vi "GetBestGuess2.vi"(9 "threshold":dbl=0.6, 10 "APIKey":string, 11 "Image":path=path "/Users/crogers/Desktop/AllThingsLEGO/AI/Ziyi/imageTest") -> (1 "score":dbl, 2 "class":string, 3 "All Data":T1)   [LabVIEW 2019]
uses:
  <vilib>/httpClient/MultipartData.ctl
  <vilib>/httpClient/LabVIEWHTTPClient.lvlib
panel:
  out "Body":string
  out "Headers":string="\r\n\r\n"
  out "error out":errorcluster
  out "Most likely":cluster{"score":dbl, "class":string}[](array[cluster])
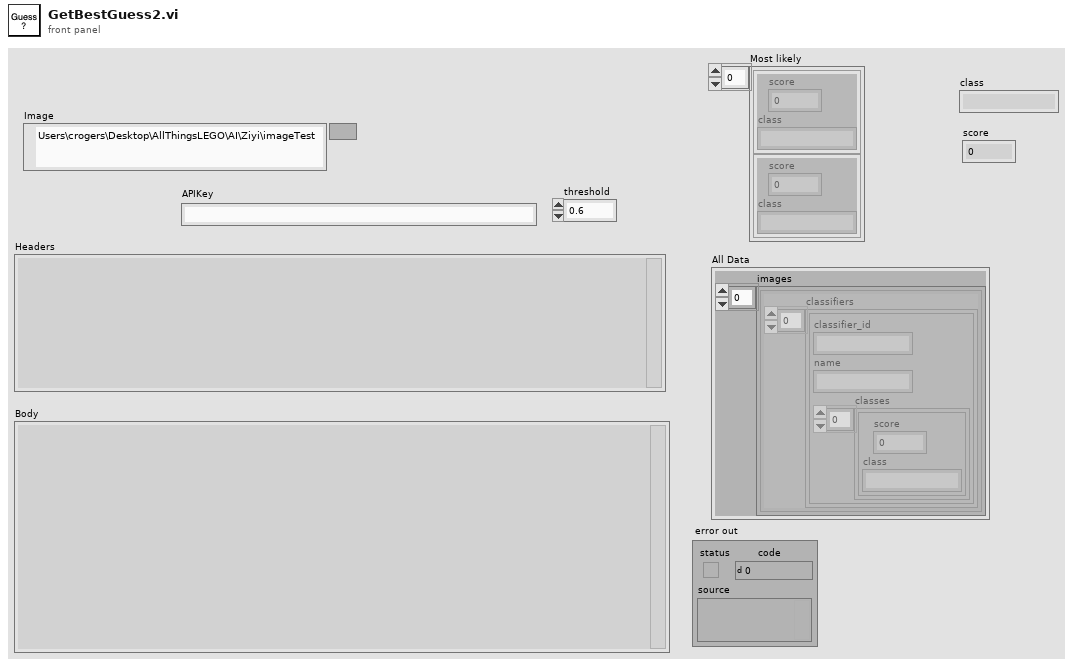
[diagram p1: front panel]
types:
  T1 = cluster{"images":cluster{"classifiers":cluster{"classifier_id":string, "name":string, "classes":cluster{"score":dbl, "class":string}[]}[]}[]}
  T2 = typedef "LabVIEWHTTPClient.lvlib/MultipartData.ctl" = cluster{"Name":string, "Value":string, "File":path, "Filename":string, "MIME type":string}
  T3 = typedef "LabVIEWHTTPClient.lvlib/ClientHandle.ctl" = refnum<k1>
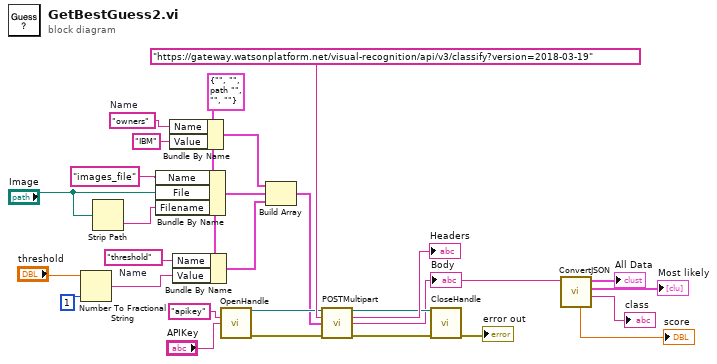
[diagram p0: block diagram]
diagram:
  w7 = "threshold"  # Name
  w2 = T2 {"Name"="", "Value"="", "File"=path "", "Filename"="", "MIME type"=""} ("Element")
  w18 = "owners"  # Name
  n1 = Number To Fractional String(number="threshold", precision (6)=i16 1 ("width (-)")) -> (F-format string=w3:string)  [unwired: 2 in]
  n2 = Strip Path(path="Image") -> (name=w10:string)  [unwired: 1 out]
  n3 = Bundle By Name(cluster=w2, "Name"="images_file" ("resulting string"), "File"="Image", "Filename"=w10) -> (w13:T2)
  n4 = Bundle By Name(cluster=w2, "Name"=w18, "Value"="IBM") -> (w17:T2)
  n5 = Bundle By Name(cluster=w2, "Name"=w7, "Value"=w3) -> (w6:T2)
  n6 = call <vilib>:"OpenHandle.vi"("username"="apikey", "password"="APIKey") -> ("client handle out"=w22:T3, "error out"=w21:errorcluster)  [unwired: 12 in]
  n7 = Build Array(w17, w13, w6) -> (w16:T2[])
  n8 = call <vilib>:"POSTMultipart.vi"("client handle"=w22, "url"="https://gateway.watsonplatform.net/visual-recognition/api/v3/classify?version=2018-03-19", "data"=w16, "error in (no error)"=w21) -> ("client handle out"=w20:T3, "headers"=→"Headers":string, "body"=w1:string, "error out"=w19:errorcluster)  [unwired: 8 in]
  "Body" <- w1
  n9 = call <vilib>:"CloseHandle.vi"("client handle"=w20, "error in (no error)"=w19) -> ("error out"=→"error out":errorcluster)  [unwired: 13 in]
  n10 = call "ConvertJSON.vi"("standard output"=w1) -> ("class"=→"class":string, "Most lik"=→"Most likely":cluster{"score":dbl, "class":string}[], "All Data"=→"All Data":T1, "score"=→"score":dbl)  [unwired: 7 in]
